vi "GOOP_LVClass_Item_OnPopUpMenu.vi"(11 "Object":u64) -> ()   [LabVIEW 2014]
uses:
  <resource>/Framework/Providers/API/mxLvMenuItem.ctl
  <resource>/Framework/Providers/Open_GDS/ClassProviders/Provider_EndevoGOOP300/EndevoProviderName.ctl
  <resource>/Framework/Providers/Open_GDS/ClassProviders/Provider_EndevoGOOP400/EndevoG4ProviderName.ctl
  <resource>/Framework/Providers/Open_GDS/ClassProviders/Common/LvClass_class/GDSLvClass_ClassTypeSettingNames.ctl
  <resource>/Framework/Providers/Open_GDS/ClassProviders/Common/ScriptingFunctions/Scripting_ConnectorPanePatternType.ctl
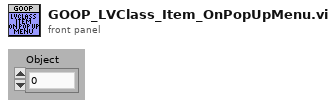
[diagram p1: front panel]
types:
  T1 = typedef "mxLvMenuItem.ctl" = cluster{"Menu Name":string, "Description":string, "Icon File Name":path, "Menu Tag":string, "Enabled":bool, "Checked":bool, "Separator":bool, "Batchable":bool, "Weight":i32, "Batch Mode (Ignored if Not Batchable)":enum32{"Show If All Items Support Command", "Show If Any Items Support Command"}, "Menu Location":enum32{"<None>", "Project", "Project / Build Specifications", "Tools", "Tools / Source Control", "Tools / Real-Time Module", "Help"}, "Exclude From Getting Started Window Menu":bool}
  T2 = typedef "EndevoG4ProviderName.ctl" = enum16{"EndevoGOOP400"}
  T3 = typedef "EndevoProviderName.ctl" = enum16{"EndevoGOOP300"}
  T4 = typedef "GDSLvClass_ClassTypeSettingNames.ctl" = enum16{"EndevoGOOP_ClassProvider", "EndevoGOOP_TemplateUsed", "EndevoGOOP_TemplateVersion", "EndevoGOOP_PlugIns", "EndevoGOOP_ConnectorPanePattern"}
  T5 = typedef "Scripting_ConnectorPanePatternType.ctl" = u16
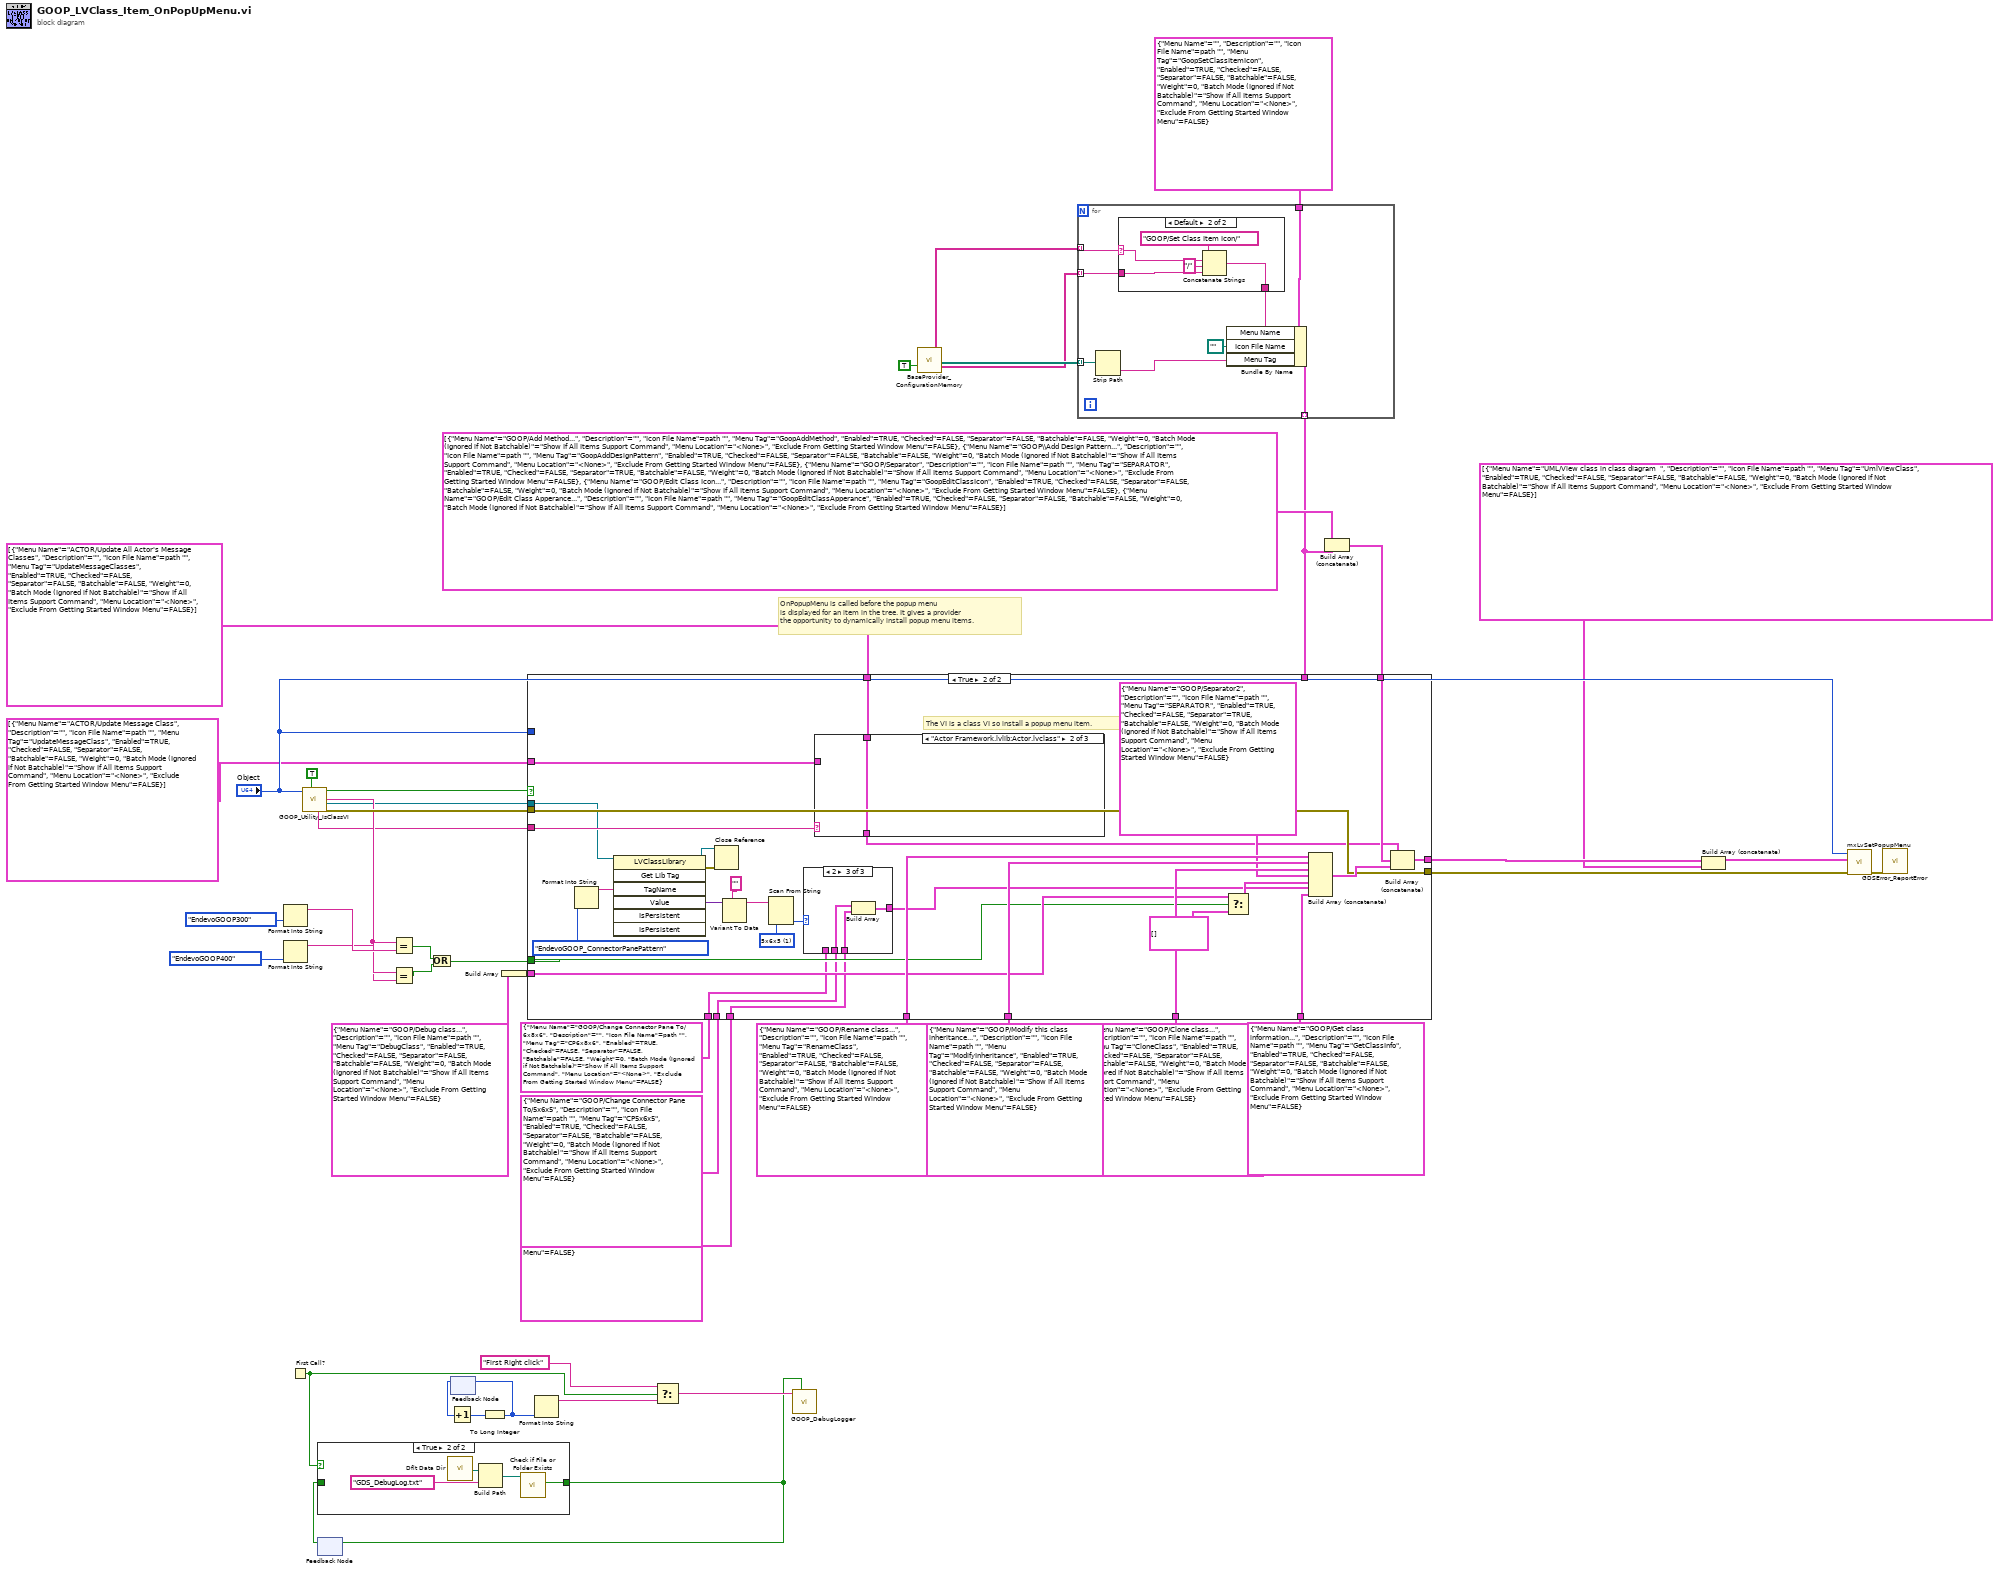
[diagram p0: block diagram]
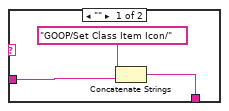
[diagram p3: hidden frame]
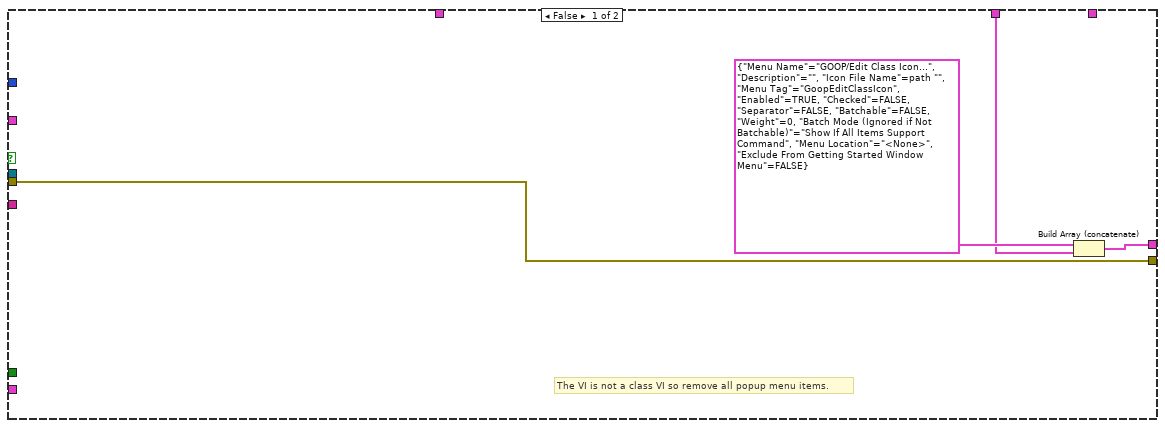
[diagram p4: hidden frame]
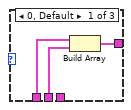
[diagram p5: hidden frame]
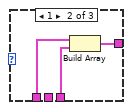
[diagram p6: hidden frame]
diagram:
  # "OnPopupMenu is called before the popup menu\nis displayed for an item in the tree. It gives a provider\nthe opportunity to dynamically install popup menu items."
  n1 = Format Into String(EndevoProviderName."EndevoGOOP300" ("ProviderName")) -> (resulting string=w26:string)  [unwired: 3 in, 1 out]
  n2 = Format Into String(EndevoG4ProviderName."EndevoGOOP400" ("ProviderName")) -> (resulting string=w23:string)  [unwired: 3 in, 1 out]
  n3 = First Call?() -> (First Call?: T/F=w11:bool)
  n4 = call <resource>:"GOOP_Utility_IsClassVI.vi"("KeepClassOpen(False)"=TRUE, "Object"="Object") -> ("error out"=w46:errorcluster, "ClassItem(If Found)"=w4:refnum<vi>, "ClassProvider"=w24:string, "Is Class VI?"=w43:bool, "RootClassQualified Class Name"=w9:string)  [unwired: 5 in]
  n5 = feedback #1() -> (w12:bool)  [unwired: 1 in]
  n6 = case shown="True" w11 {
    tunnel: [w48 w49] -> w10
    tunnel: w12 -> [w48 _]
    frame False {
    }
    frame True {
      n7 = call <vilib>:"Dflt Data Dir.vi"() -> ("App:Default Data Directory"=w51:path)
      n8 = Build Path(base path=w51, name or relative path="GDS_DebugLog.txt") -> (appended path=w52:path)
      n9 = call <vilib>:"Check if File or Folder Exists.vi"("path"=w52) -> ("file or folder exists?"=w49:bool)  [unwired: 8 in, 2 out]
    }
  }
  n10 = feedback-in #1(w10) -> ()
  n11 = Equal?(x=w24, y=w26) -> (x = y?=w21:bool)
  n12 = Equal?(x=w24, y=w23) -> (x = y?=w22:bool)
  n13 = Or(x=w21, y=w22) -> (x .or. y?=w20:bool)
  n14 = feedback #2() -> (w16:i32)  [unwired: 1 in]
  n15 = Increment(x=w16) -> (x+1=w15:i32)
  n16 = To Long Integer(number=w15) -> (32bit integer=w14:i32)
  n17 = feedback-in #2(w14) -> ()
  n18 = Build Array(T1 {"Menu Name"="GOOP/Debug class...", "Description"="", "Icon File Name"=path "", "Menu Tag"="DebugClass", "Enabled"=TRUE, "Checked"=FALSE, "Separator"=FALSE, "Batchable"=FALSE, "Weight"=0, "Batch Mode (Ignored if Not Batchable)"=enum."Show If All Items Support Command", "Menu Location"=enum."<None>", "Exclude From Getting Started Window Menu"=FALSE} ("Menu Item")) -> (w27:T1[])
  n19 = Format Into String(w14) -> (resulting string=w13:string)  [unwired: 3 in, 1 out]
  n20 = Select(t="First Right click" ("name or relative path"), s=w11, f=w13) -> (s? t:f=w18:string)
  n21 = call <resource>:"GOOP_DebugLogger.vi"("ActivateDebugging"=w10, "State"=w18) -> ()  [unwired: 8 in, 2 out]
  n22 = call <resource>:"BaseProvider_ConfigurationMemory.vi"("Filter_Icons"=TRUE) -> ("ClassItemIconGroup"=w19:string[], "ClassItemIconPaths"=w30:path[], "ClassItemIconNames"=w29:string[])  [unwired: 12 in, 4 out]
  n23 = for {
    tunnel: [w59] -> w32 mode=indexing
    tunnel: T1 {"Menu Name"="", "Description"="", "Icon File Name"=path "", "Menu Tag"="GoopSetClassItemIcon", "Enabled"=TRUE, "Checked"=FALSE, "Separator"=FALSE, "Batchable"=FALSE, "Weight"=0, "Batch Mode (Ignored if Not Batchable)"=enum."Show If All Items Support Command", "Menu Location"=enum."<None>", "Exclude From Getting Started Window Menu"=FALSE} ("Menu Item") -> [w60]
    tunnel: w30 -> [w56] mode=indexing
    tunnel: w29 -> [w54] mode=indexing
    tunnel: w19 -> [w53] mode=indexing
    n24 = Strip Path(path=w56) -> (name=w55:string)  [unwired: 1 out]
    n25 = case shown="Default" w53 {
      selector: w53 -> [_ w65]
      tunnel: [w62 w68] -> w57
      tunnel: w54 -> [w61 w67]
      frame "" {
        n26 = Concatenate Strings("GOOP/Set Class Item Icon/" ("string"), w61) -> (w62:string)
      }
      frame Default {
        n27 = Concatenate Strings("GOOP/Set Class Item Icon/" ("string"), w65, "/" ("string"), w67) -> (w68:string)
      }
    }
    n28 = Bundle By Name(cluster=w60, "Menu Name"=w57, "Icon File Name"=path "", "Menu Tag"=w55) -> (w59:T1)
  }
  n29 = Build Array (concatenate)(T1[] [{"Menu Name"="GOOP/Add Method...", "Description"="", "Icon File Name"=path "", "Menu Tag"="GoopAddMethod", "Enabled"=TRUE, "Checked"=FALSE, "Separator"=FALSE, "Batchable"=FALSE, "Weight"=0, "Batch Mode (Ignored if Not Batchable)"=enum."Show If All Items Support Command", "Menu Location"=enum."<None>", "Exclude From Getting Started Window Menu"=FALSE}, {"Menu Name"="GOOP\\Add Design Pattern...", "Description"="", "Icon File Name"=path "", "Menu Tag"="GoopAddDesignPattern", "Enabled"=TRUE, "Checked"=FALSE, "Separator"=FALSE, "Batchable"=FALSE, "Weight"=0, "Batch Mode (Ignored if Not Batchable)"=enum."Show If All Items Support Command", "Menu Location"=enum."<None>", "Exclude From Getting Started Window Menu"=FALSE}, {"Menu Name"="GOOP/Separator", "Description"="", "Icon File Name"=path "", "Menu Tag"="SEPARATOR", "Enabled"=TRUE, "Checked"=FALSE, "Separator"=TRUE, "Batchable"=FALSE, "Weight"=0, "Batch Mode (Ignored if Not Batchable)"=enum."Show If All Items Support Command", "Menu Location"=enum."<None>", "Exclude From Getting Started Window Menu"=FALSE}, {"Menu Name"="GOOP/Edit Class Icon...", "Description"="", "Icon File Name"=path "", "Menu Tag"="GoopEditClassIcon", "Enabled"=TRUE, "Checked"=FALSE, "Separator"=FALSE, "Batchable"=FALSE, "Weight"=0, "Batch Mode (Ignored if Not Batchable)"=enum."Show If All Items Support Command", "Menu Location"=enum."<None>", "Exclude From Getting Started Window Menu"=FALSE}, {"Menu Name"="GOOP/Edit Class Apperance...", "Description"="", "Icon File Name"=path "", "Menu Tag"="GoopEditClassApperance", "Enabled"=TRUE, "Checked"=FALSE, "Separator"=FALSE, "Batchable"=FALSE, "Weight"=0, "Batch Mode (Ignored if Not Batchable)"=enum."Show If All Items Support Command", "Menu Location"=enum."<None>", "Exclude From Getting Started Window Menu"=FALSE}], w32) -> (w33:T1[])
  n30 = case shown="True" w43 {
    tunnel: [w70 w102] -> w42
    tunnel: "Object" -> [_ _]
    tunnel: w46 -> [w72 w91]
    tunnel: w4 -> [_ w83]
    tunnel: T1 {"Menu Name"="GOOP/Modify this class inheritance...", "Description"="", "Icon File Name"=path "", "Menu Tag"="ModifyInheritance", "Enabled"=TRUE, "Checked"=FALSE, "Separator"=FALSE, "Batchable"=FALSE, "Weight"=0, "Batch Mode (Ignored if Not Batchable)"=enum."Show If All Items Support Command", "Menu Location"=enum."<None>", "Exclude From Getting Started Window Menu"=FALSE} ("Menu Item") -> [_ w100]
    tunnel: [w72 w91] -> w5
    tunnel: w33 -> [_ w101]
    tunnel: T1 {"Menu Name"="GOOP/Get class information...", "Description"="", "Icon File Name"=path "", "Menu Tag"="GetClassInfo", "Enabled"=TRUE, "Checked"=FALSE, "Separator"=FALSE, "Batchable"=FALSE, "Weight"=0, "Batch Mode (Ignored if Not Batchable)"=enum."Show If All Items Support Command", "Menu Location"=enum."<None>", "Exclude From Getting Started Window Menu"=FALSE} ("Menu Item") -> [_ w96]
    tunnel: T1 {"Menu Name"="GOOP/Rename class...", "Description"="", "Icon File Name"=path "", "Menu Tag"="RenameClass", "Enabled"=TRUE, "Checked"=FALSE, "Separator"=FALSE, "Batchable"=FALSE, "Weight"=0, "Batch Mode (Ignored if Not Batchable)"=enum."Show If All Items Support Command", "Menu Location"=enum."<None>", "Exclude From Getting Started Window Menu"=FALSE} ("Menu Item") -> [_ w99]
    tunnel: T1 {"Menu Name"="GOOP/Clone class...", "Description"="", "Icon File Name"=path "", "Menu Tag"="CloneClass", "Enabled"=TRUE, "Checked"=FALSE, "Separator"=FALSE, "Batchable"=FALSE, "Weight"=0, "Batch Mode (Ignored if Not Batchable)"=enum."Show If All Items Support Command", "Menu Location"=enum."<None>", "Exclude From Getting Started Window Menu"=FALSE} ("Menu Item") -> [_ w98]
    tunnel: w27 -> [_ w93]
    tunnel: w32 -> [w69 _]
    tunnel: w20 -> [_ w92]
    tunnel: w9 -> [_ w90]
    tunnel: T1[] [{"Menu Name"="ACTOR/Update All Actor's Message Classes", "Description"="", "Icon File Name"=path "", "Menu Tag"="UpdateMessageClasses", "Enabled"=TRUE, "Checked"=FALSE, "Separator"=FALSE, "Batchable"=FALSE, "Weight"=0, "Batch Mode (Ignored if Not Batchable)"=enum."Show If All Items Support Command", "Menu Location"=enum."<None>", "Exclude From Getting Started Window Menu"=FALSE}] -> [_ w89]
    tunnel: T1[] [{"Menu Name"="ACTOR/Update Message Class", "Description"="", "Icon File Name"=path "", "Menu Tag"="UpdateMessageClass", "Enabled"=TRUE, "Checked"=FALSE, "Separator"=FALSE, "Batchable"=FALSE, "Weight"=0, "Batch Mode (Ignored if Not Batchable)"=enum."Show If All Items Support Command", "Menu Location"=enum."<None>", "Exclude From Getting Started Window Menu"=FALSE}] -> [_ w88]
    tunnel: T1 {"Menu Name"="GOOP/Change Connector Pane To/6x8x6", "Description"="", "Icon File Name"=path "", "Menu Tag"="CP6x8x6", "Enabled"=TRUE, "Checked"=FALSE, "Separator"=FALSE, "Batchable"=FALSE, "Weight"=0, "Batch Mode (Ignored if Not Batchable)"=enum."Show If All Items Support Command", "Menu Location"=enum."<None>", "Exclude From Getting Started Window Menu"=FALSE} ("Menu Item") -> [_ w75]
    tunnel: T1 {"Menu Name"="GOOP/Change Connector Pane To/5x6x5", "Description"="", "Icon File Name"=path "", "Menu Tag"="CP5x6x5", "Enabled"=TRUE, "Checked"=FALSE, "Separator"=FALSE, "Batchable"=FALSE, "Weight"=0, "Batch Mode (Ignored if Not Batchable)"=enum."Show If All Items Support Command", "Menu Location"=enum."<None>", "Exclude From Getting Started Window Menu"=FALSE} ("Menu Item") -> [_ w74]
    tunnel: T1 {"Menu Name"="GOOP/Change Connector Pane To/4x4x4", "Description"="", "Icon File Name"=path "", "Menu Tag"="CP4x4x4", "Enabled"=TRUE, "Checked"=FALSE, "Separator"=FALSE, "Batchable"=FALSE, "Weight"=0, "Batch Mode (Ignored if Not Batchable)"=enum."Show If All Items Support Command", "Menu Location"=enum."<None>", "Exclude From Getting Started Window Menu"=FALSE} ("Menu Item") -> [_ w73]
    frame False {
      # "The VI is not a class VI so remove all popup menu items."
      n31 = Build Array (concatenate)(T1 {"Menu Name"="GOOP/Edit Class Icon...", "Description"="", "Icon File Name"=path "", "Menu Tag"="GoopEditClassIcon", "Enabled"=TRUE, "Checked"=FALSE, "Separator"=FALSE, "Batchable"=FALSE, "Weight"=0, "Batch Mode (Ignored if Not Batchable)"=enum."Show If All Items Support Command", "Menu Location"=enum."<None>", "Exclude From Getting Started Window Menu"=FALSE} ("Menu Item"), w69) -> (w70:T1[])
    }
    frame True {
      w79 = T5 1 items=["4x4x4", "5x6x5", "6x8x6"] ("Pattern")
      # "The VI is a class VI so install a popup menu item."
      n32 = Format Into String(GDSLvClass_ClassTypeSettingNames."EndevoGOOP_ConnectorPanePattern" ("ClassTypeSettingNames")) -> (resulting string=w85:string)  [unwired: 3 in, 1 out]
      n33 = invoke class="LVClassLibrary" method="Get Lib Tag"(reference=w83, "TagName"=w85) -> (reference out=w81:refnum<vi>, error out=w82:errorcluster, "Value"=w86:variant)  [unwired: 5 in, 4 out]
      n34 = Close Reference(reference=w81, error in (no error)=w82) -> ()  [unwired: 1 out]
      n35 = Variant To Data(type="", Variant=w86) -> (data=w78:string)  [unwired: 1 in, 1 out]
      n36 = Scan From String(input string=w78, default 1=w79) -> (output 1=w77:T5)  [unwired: 3 in, 3 out]
      n37 = case shown="2" w77 {
        tunnel: [w106 w109 w112] -> w76
        tunnel: w75 -> [w105 w108 _]
        tunnel: w74 -> [w104 _ w110]
        tunnel: w73 -> [_ w107 w111]
        frame 0, Default {
          n38 = Build Array(w105, w104) -> (w106:T1[])
        }
        frame 1 {
          n39 = Build Array(w108, w107) -> (w109:T1[])
        }
        frame 2 {
          n40 = Build Array(w110, w111) -> (w112:T1[])
        }
      }
      n41 = case shown="\"Actor Framework.lvlib:Actor.lvclass\"" w90 {
        tunnel: w89 -> [_ w113 _]
        tunnel: [_ w113 w114] -> w87
        tunnel: w88 -> [_ _ w114]
        frame Default {
        }
        frame "Actor Framework.lvlib:Actor.lvclass" {
        }
        frame "Actor Framework.lvlib:Message.lvclass" {
        }
      }
      n42 = Select(t=w93, s=w92, f=T1[] []) -> (s? t:f=w95:T1[])
      n43 = Build Array (concatenate)(w99, w100, w98, T1 {"Menu Name"="GOOP/Separator2", "Description"="", "Icon File Name"=path "", "Menu Tag"="SEPARATOR", "Enabled"=TRUE, "Checked"=FALSE, "Separator"=TRUE, "Batchable"=FALSE, "Weight"=0, "Batch Mode (Ignored if Not Batchable)"=enum."Show If All Items Support Command", "Menu Location"=enum."<None>", "Exclude From Getting Started Window Menu"=FALSE} ("Menu Item"), w95, w76, w96) -> (w103:T1[])
      n44 = Build Array (concatenate)(w87, w101, w103) -> (w102:T1[])
    }
  }
  n45 = Build Array (concatenate)(w42, T1[] [{"Menu Name"="UML/View class in class diagram  ", "Description"="", "Icon File Name"=path "", "Menu Tag"="UmlViewClass", "Enabled"=TRUE, "Checked"=FALSE, "Separator"=FALSE, "Batchable"=FALSE, "Weight"=0, "Batch Mode (Ignored if Not Batchable)"=enum."Show If All Items Support Command", "Menu Location"=enum."<None>", "Exclude From Getting Started Window Menu"=FALSE}]) -> (w41:T1[])
  n46 = call <resource>:"mxLvSetPopupMenu.vi"("error in"=w5, "Popup Menu Items"=w41, "Item"="Object") -> ("error out"=w37:errorcluster)  [unwired: 7 in, 1 out]
  n47 = call <resource>:"GDSError_ReportError.vi"("error in (no error)"=w37) -> ()  [unwired: 18 in, 1 out]
